vi "File_path.vi"(8 "error in (no error)":errorcluster, 10 "Path":path, 11 "Contador_Bin_Actor in":refnum<class "Contador_Bin_Actor.lvclass">) -> (0 "error out":errorcluster, 3 "Contador_Bin_Actor out":refnum<class "Contador_Bin_Actor.lvclass">)   [LabVIEW 2019, in "Contador_Bin_Actor.lvlib" / "Contador_Bin_Actor.lvclass"]
uses:
  Contador_Bin_Actor.lvclass
  Contador_Bin_Actor.lvclass/Contador_Bin_Actor.ctl
  Logging_Contador_Actor/Logging_Contador_Actor Messages/Write Path Msg/Write Path Msg.lvclass/Write Path Msg.ctl
  <vilib>/ActorFramework/Message Enqueuer/Message Enqueuer.lvclass/Message Enqueuer.ctl
  <vilib>/ActorFramework/Message Enqueuer/Enqueue.vi
  Logging_Contador_Actor/Logging_Contador_Actor Messages/Write Path Msg/Write Path Msg.lvclass
  C:/Program Files/National Instruments/LabVIEW 2019/vi.lib/ActorFramework/Message/Message.lvclass
  <vilib>/ActorFramework/Message Priority Queue/Priority Enqueue.vi
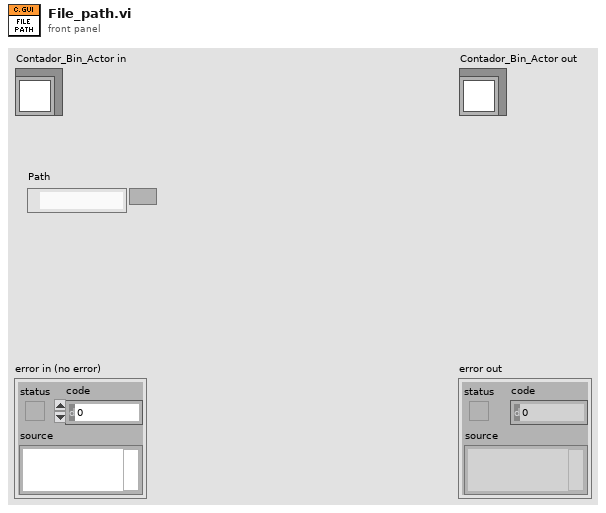
[diagram p1: front panel]
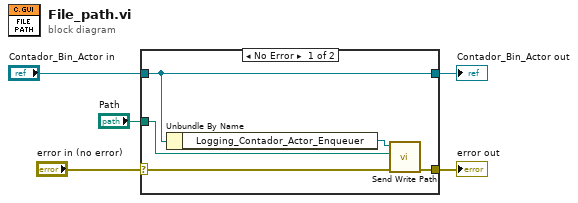
[diagram p0: block diagram]
diagram:
  n1 = case shown="No Error" "error in (no error)" {
    selector: "error in (no error)" -> [w7 w12]
    tunnel: [w6 w12] -> w4
    tunnel: [w9 w11] -> w2
    tunnel: "Contador_Bin_Actor in" -> [w9 w11]
    tunnel: "Path" -> [w10 _]
    frame No Error {
      n2 = Unbundle By Name(w9) -> ("Logging_Contador_Actor_Enqueuer"=w8:refnum<class "Message Enqueuer.lvclass">)
      n3 = call "Send Write Path.vi"("error in (no error)"=w7, "Path"=w10, "Message Enqueuer"=w8) -> ("error out"=w6:errorcluster)  [unwired: 7 in, 1 out]
    }
    frame Error {
    }
  }
  "error out" <- w4
  "Contador_Bin_Actor out" <- w2
